vi "Global FIFO variabls.vi"() -> ()   [LabVIEW 2012]
panel:
  out "Stop SPC Read":bool
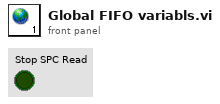
[diagram p1: front panel]
diagram:
